vi "simple_foo_call.vi"() -> ()   [LabVIEW 2018]
panel:
  out "outputs":string[](array[string])
  out "output":string
  out "appended path":path
  out "error out":errorcluster
  in  "error in (no error)":errorcluster
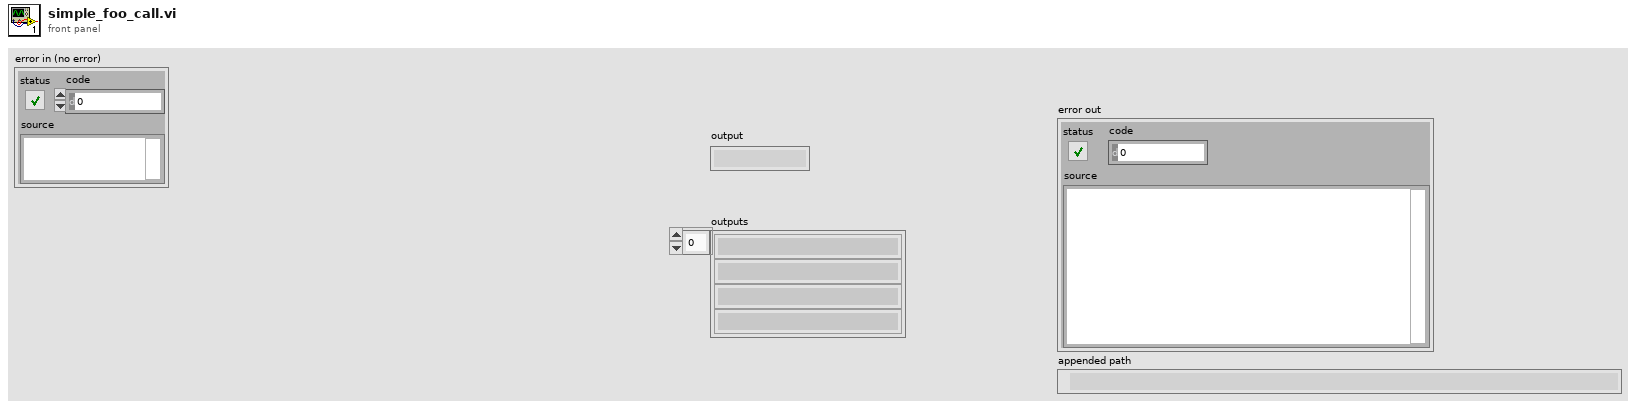
[diagram p1: front panel]
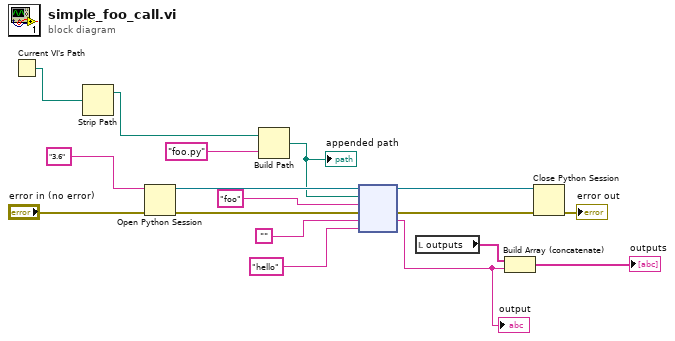
[diagram p0: block diagram]
diagram:
  n1 = Current VI's Path() -> (path=w4:path)
  n2 = Strip Path(path=w4) -> (stripped path=w3:path)  [unwired: 1 out]
  n3 = Open Python Session(python version="3.6" ("Python version"), 3:"error in (no error)") -> (session out=w14:refnum<k35>, error out=w16:errorcluster)  [unwired: 1 in]
  n4 = Build Path(base path=w3, name or relative path="foo.py") -> (appended path=w7:path)
  "appended path" <- w7
  n5 = node(w14, w7, "foo" ("function name"), w16, "", "hello") -> (w13:refnum<k35>, w15:errorcluster, w2:string)  [unwired: 1 in, 2 out]
  "output" <- w2
  n6 = local read "outputs"() -> (w10:string[])
  n7 = Build Array (concatenate)(w10, w2) -> (→"outputs":string[])
  n8 = Close Python Session(session in=w13, error in=w15) -> (11:→"error out":errorcluster)
